vi "Rio_Main.vi"() -> ()   [LabVIEW 2015]
doc: "The myRIO Project template acquires acceleration data from the onboard accelerometer and displays the changes of acceleration values in a waveform chart."
panel:
  out "Current Angle":i32
  in  "Desired Angle (Deg)":i32 min=-90 max=90 step=1
  in  "Stop Button":bool
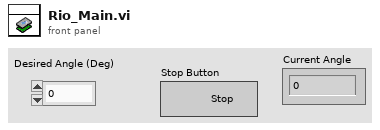
[diagram p1: front panel]
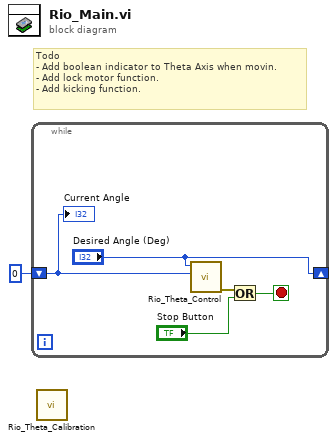
[diagram p0: block diagram]
diagram:
  # "Todo\n- Add boolean indicator to Theta Axis when movin.\n- Add lock motor function.\n- Add kicking function."
  n1 = while {
    shift-right: ["Desired Angle (Deg)"] -> _
    shift-left: 0 ("Desired Angle (Deg)") -> [w4]
    stop <- w3 stop-if-true
    n2 = call "Rio_Theta_Control.vi"("Current Angle (Deg)"=w4, "Desired Angle (Deg)"="Desired Angle (Deg)") -> ("error out"=w2:errorcluster)  [unwired: 8 in, 1 out]
    n3 = Or(x=w2, y="Stop Button") -> (x .or. y?=w3:bool)
    "Current Angle" <- w4
  }
  n4 = call "Rio_Theta_Calibration.vi"() -> ()  [unwired: 10 in, 2 out]
